vi "arduinoInit.vi"(1 "valve open time":u32=1000, 2 "baud rate":u32=57600, 3 "USB COM port":refnum<visa-resource-name>="COM4") -> (0 "serial status":u32(colorbox)=6618880)   [LabVIEW 2012]
uses:
  GlobalArduino.vi
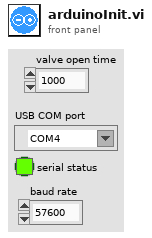
[diagram p1: front panel]
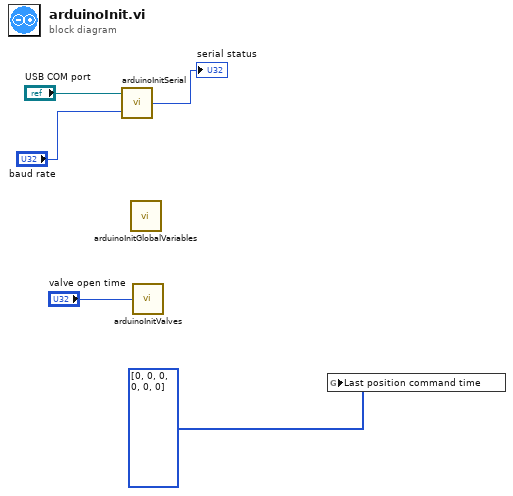
[diagram p0: block diagram]
diagram:
  n1 = call "arduinoInitSerial.vi"("Serial Settings:Baud Rate"="baud rate", "VISA resource name"="USB COM port") -> ("serial status"=→"serial status":u32)
  n2 = call "arduinoInitGlobalVariables.vi"() -> ()  [unwired: 12 in]
  n3 = call "arduinoInitValves.vi"("valve open time"="valve open time") -> ()
  n4 = global write "GlobalArduino.vi" "Last position command time"(u64[] [0, 0, 0, 0, 0, 0] ("Last position command time")) -> ()
